vi "temp.vi"() -> ()   [LabVIEW 2019]
panel:
  in  "Fit axis(0:xaxis, 1:yaxis)":i32=1
  out "regressionSigma":dbl[](array[numeric])
  out "regressionTime":dbl[](array[numeric])
  in  "rcropsize":i32=100
  in  "rcropy":i32=480
  in  "rcropx":i32=460
  in  "cropsize":i32=350
  in  "cropy":i32=500
  in  "cropx":i32=770
  out "Temperature(K)":dbl
  out "sigma":dbl[](array[numeric])
  out "time(ms)":dbl[](array[numeric])
  in  "BG":string="C:\\Users\\Yuan Yujia\\Desktop\\mottof\\bg.jpg"
  in  "function name":string="temperature"
  in  "Python version":string="3.8.2"
  in  "module path":path=path "C:/Users/Yuan Yujia/Desktop/mottof/MOTTOF3.py"
  in  "Image":string[](array[string])=["C:\\Users\\Yuan Yujia\\Desktop\\mottof\\05000us_0.jpg", "C:\\Users\\Yuan Yujia\\Desktop\\mottof\\07000us_0.jpg", "C:\\Users\\Yuan Yujia\\Desktop\\mottof\\09000us_0.jpg", "C:\\Users\\Yuan Yujia\\Desktop\\mottof\\11000us_0.jpg", "C:\\Users\\Yuan Yujia\\Desktop\\mottof\\13000us_0.jpg", "C:\\Users\\Yuan Yujia\\Desktop\\mottof\\15000us_0.jpg", "C:\\Users\\Yuan Yujia\\Desktop\\mottof\\17000us_0.jpg", "C:\\Users\\Yuan Yujia\\Desktop\\mottof\\19000us_0.jpg", "C:\\Users\\Yuan Yujia\\Desktop\\mottof\\21000us_0.jpg"]
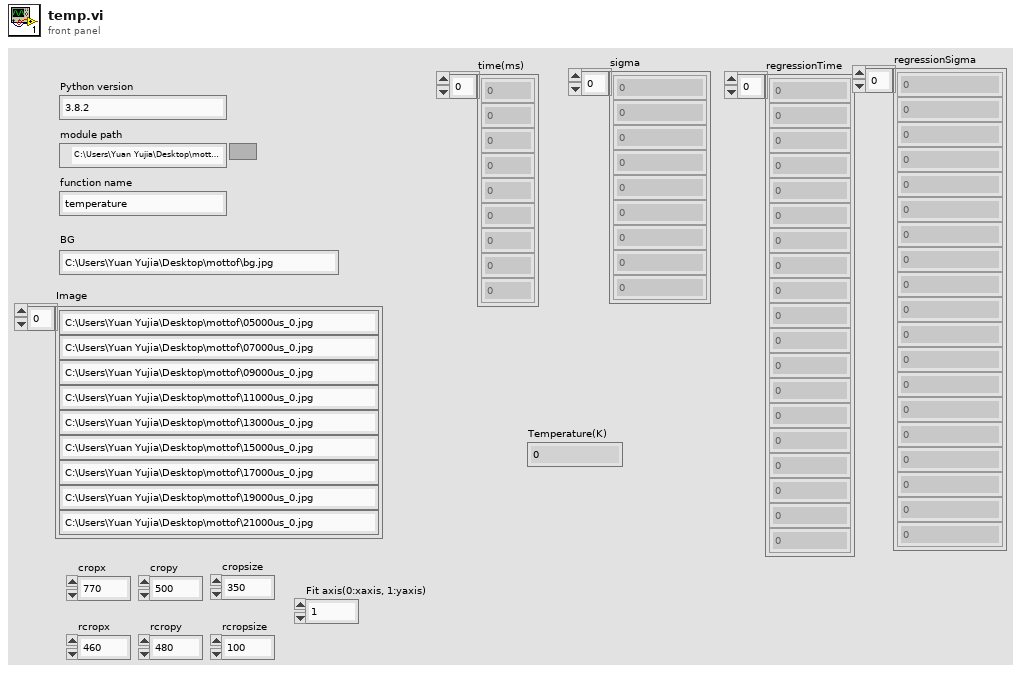
[diagram p1: front panel]
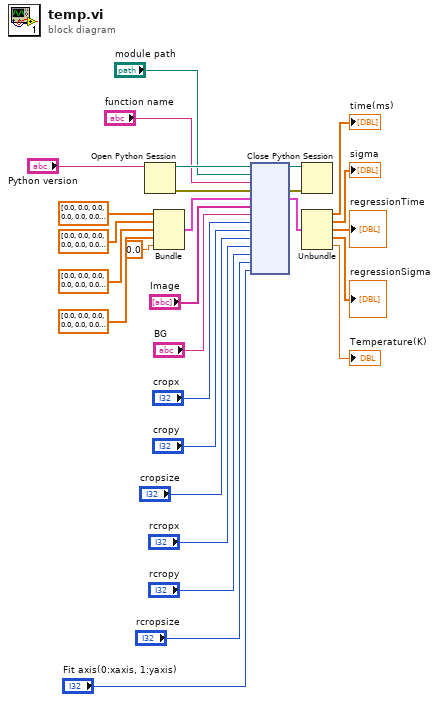
[diagram p0: block diagram]
diagram:
  n1 = Open Python Session(python version="Python version") -> (session out=w28:refnum<k35>, error out=w27:errorcluster)  [unwired: 2 in]
  n2 = Bundle(dbl[] [0.0, 0.0, 0.0, 0.0, 0.0, 0.0, 0.0, 0.0, 0.0], dbl[] [0.0, 0.0, 0.0, 0.0, 0.0, 0.0, 0.0, 0.0, 0.0], dbl[] [0.0, 0.0, 0.0, 0.0, 0.0, 0.0, 0.0, 0.0, 0.0], dbl[] [0.0, 0.0, 0.0, 0.0, 0.0, 0.0, 0.0, 0.0, 0.0], 0.0) -> (w17:cluster{dbl[], dbl[], dbl[], dbl[], dbl})  [unwired: 1 in]
  n3 = node(w28, "module path", "function name", w27, w17, "Image", "BG", "cropx", "cropy", "cropsize", "rcropx", "rcropy", "rcropsize", "Fit axis(0:xaxis, 1:yaxis)") -> (w23:refnum<k35>, w22:errorcluster, w16:cluster{dbl[], dbl[], dbl[], dbl[], dbl})  [unwired: 9 in, 2 out]
  n4 = Close Python Session(session in=w23, error in=w22) -> ()  [unwired: 1 out]
  n5 = Unbundle(w16) -> (→"time(ms)":dbl[], →"sigma":dbl[], →"regressionTime":dbl[], →"regressionSigma":dbl[], →"Temperature(K)":dbl)
